vi "dummy_data _check.vi"() -> ()   [LabVIEW 2014]
panel:
  in  "Cmd type":i32
  out "error out":errorcluster
  in  "error in (no error)":errorcluster
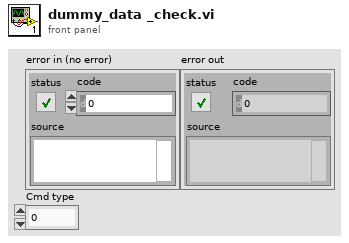
[diagram p1: front panel]
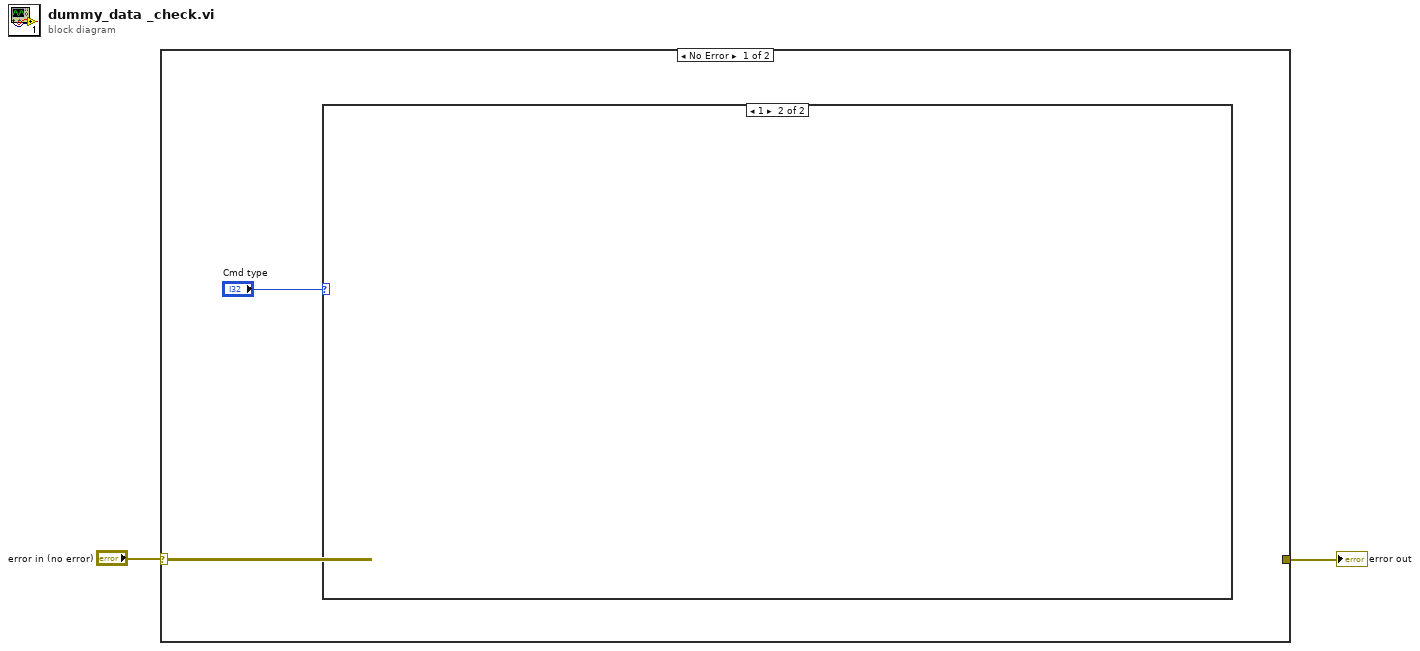
[diagram p0: block diagram]
diagram:
  n1 = case shown="No Error" "error in (no error)" {
    selector: "error in (no error)" -> [_ w4]
    tunnel: [_ w4] -> w1
    frame No Error {
      n2 = case shown="1" "Cmd type" {
        frame 0, Default {
        }
        frame 1 {
        }
      }
    }
    frame Error {
    }
  }
  "error out" <- w1
